vi "Set TDMS logfile.vi"(7 "TDMS Module Alias":string, 8 "log name":string, 9 "Log Directory":string, 10 "Config File Save Path":path, 11 "Config File Path":path) -> (0 "error out":errorcluster)   [LabVIEW 2014]
doc: "Update the log file a TDMS module will write to"
uses:
  <vilib>/NI/DCAF/Modules/TDMS Datalogger/configuration/TDMS datalogger configuration.lvclass
  <vilib>/NI/DCAF/Modules/TDMS Datalogger/configuration/TDMS datalogger configuration.lvclass/TDMS datalogger configuration.ctl
  <vilib>/NI/Configuration Framework/tree serializer/NISE_CEF_TreeSerializer.lvlib
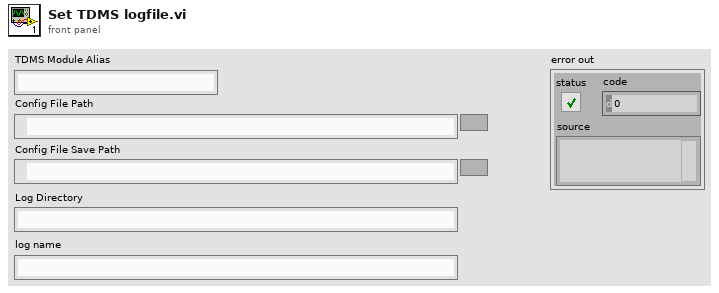
[diagram p1: front panel]
types:
  T1 = typedef "NISE_CEF_TreeSerializer.lvlib/base file format.ctl" = cluster{"version":string, "data":string}
  T2 = typedef "NISE_CEF_TreeSerializer.lvlib/flat hierarchy.ctl" = cluster{"hierarchy structure":T3, "instance data":T5[]}
  T3 = typedef "NISE_CEF_TreeSerializer.lvlib/full hierarchy.ctl" = cluster{"root":string, "hierarchy":T4[]}
  T4 = typedef "NISE_CEF_TreeSerializer.lvlib/hierarchy element.ctl" = cluster{"current node":string, "children":string[]}
  T5 = typedef "NISE_CEF_TreeSerializer.lvlib/instance data.ctl" = cluster{"ID":string, "Alias":string, "class":string, "version":string, "data":string}
  T6 = typedef "NISE_CEF_TreeSerializer.lvlib/memory hierarchy.ctl" = cluster{"hierarchy structure":T3, "instance data":refnum<class "NISE_CEF_serializable configuration.lvclass">[]}
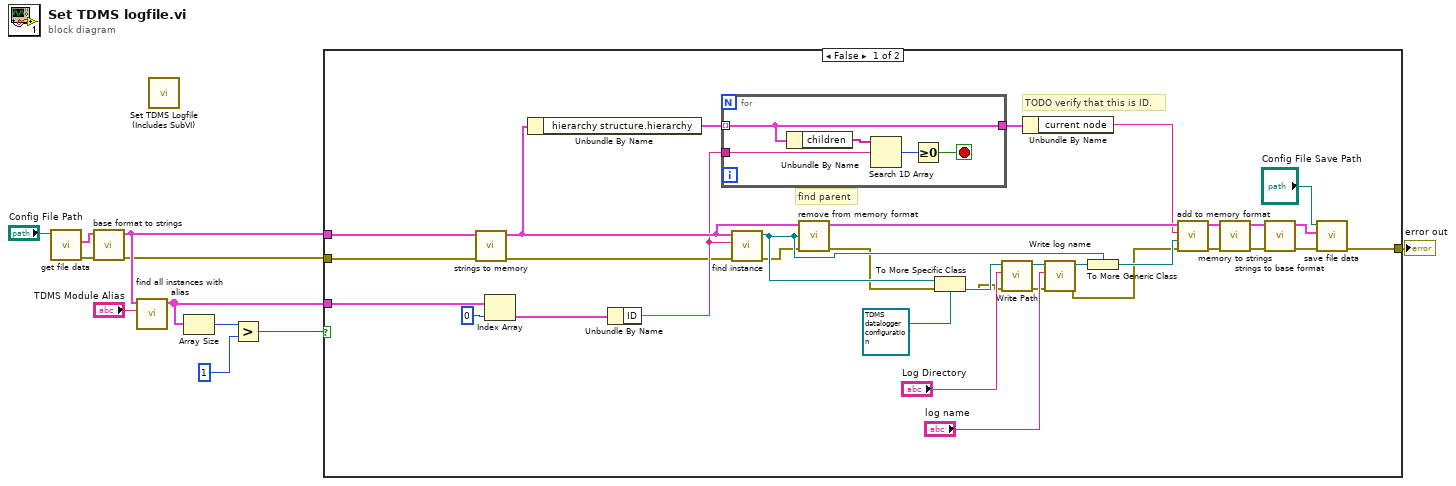
[diagram p0: block diagram]
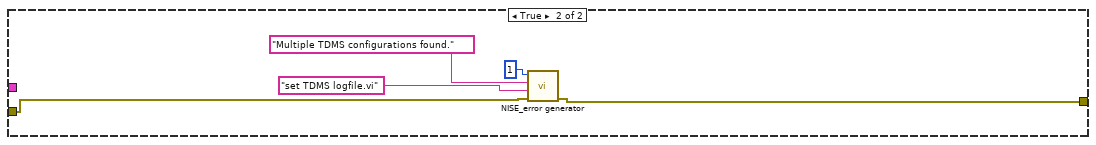
[diagram p2: hidden frame]
diagram:
  n1 = call <vilib>:"get file data.vi"("Path"="Config File Path") -> ("error out"=w11:errorcluster, "format"=w10:T1)  [unwired: 9 in]
  n2 = call <vilib>:"base format to strings.vi"("error in"=w11, "format"=w10) -> ("error out"=w5:errorcluster, "data"=w7:T2)  [unwired: 8 in]
  n3 = call <vilib>:"find all instances with alias.vi"("Alias"="TDMS Module Alias", "flat hierarchy"=w7) -> ("instance data"=w4:T5[])  [unwired: 9 in]
  n4 = call "Set TDMS Logfile (Includes SubVI).vi"() -> ()  [unwired: 12 in]
  n5 = Array Size(array=w4) -> (size(s)=w3:i32)
  n6 = Greater?(x=w3, y=1) -> (0:w1:bool)
  n7 = case shown="False" w1 {
    tunnel: w7 -> [w40 _]
    tunnel: [w19 w50] -> w6
    tunnel: w5 -> [w17 w51]
    tunnel: w4 -> [w12 _]
    frame False {
      # "TODO verify that this is ID."
      # "find parent"
      n8 = call <vilib>:"strings to memory.vi"("error in"=w17, "1.0.0"=w40) -> ("error out"=w16:errorcluster, "memory hierarchy"=w26:T6)  [unwired: 8 in]
      n9 = Index Array(array=w12, index=0) -> (element=w41:T5)
      n10 = Unbundle By Name(w26) -> ("hierarchy structure.hierarchy"=w25:T4[])
      n11 = Unbundle By Name(w41) -> ("ID"=w24:string)
      n12 = for {
        tunnel: w25 -> [w47] mode=indexing
        tunnel: w24 -> [w48]
        tunnel: [w47] -> w23
        stop <- w45 stop-if-true
        n13 = Unbundle By Name(w47) -> ("children"=w49:string[])
        n14 = Search 1D Array(1D array=w49, element=w48) -> (index of element=w46:i32)  [unwired: 1 in]
        n15 = Greater Or Equal To 0?(x=w46) -> (x >= 0?=w45:bool)
      }
      n16 = call <vilib>:"find instance.vi"("error in"=w16, "ID"=w24, "memory hierarchy"=w26) -> ("error out"=w14:errorcluster, "configuration"=w28:refnum<class "NISE_CEF_serializable configuration.lvclass">)  [unwired: 7 in]
      n17 = call <vilib>:"remove from memory format.vi"("error in"=w14, "NISE_CEF_serializable configuration in"=w28, "memory hierarchy in"=w26) -> ("error out"=w13:errorcluster, "memory hierarchy out"=w27:T6)  [unwired: 7 in]
      n18 = To More Specific Class(target class=refnum<class "TDMS datalogger configuration.lvclass"> refnum ("TDMS datalogger configuration"), reference=w28, error in=w13) -> (specific class reference=w39:refnum<class "TDMS datalogger configuration.lvclass">, error out=w35:errorcluster)
      n19 = call <vilib>:"Write Path.vi"("error in (no error)"=w35, "Log Directory"="Log Directory", "TDMS datalogger configuration in"=w39) -> ("error out"=w34:errorcluster, "TDMS datalogger configuration out"=w37:refnum<class "TDMS datalogger configuration.lvclass">)  [unwired: 7 in]
      n20 = Unbundle By Name(w23) -> ("current node"=w22:string)
      n21 = call <vilib>:"Write log name.vi"("error in (no error)"=w34, "log name"="log name", "TDMS datalogger configuration in"=w37) -> ("error out"=w15:errorcluster, "TDMS datalogger configuration out"=w33:refnum<class "TDMS datalogger configuration.lvclass">)  [unwired: 7 in]
      n22 = To More Generic Class(target class=w28, reference=w33) -> (generic class reference=w29:refnum<class "NISE_CEF_serializable configuration.lvclass">)
      n23 = call <vilib>:"add to memory format.vi"("error in"=w15, "NISE_CEF_serializable configuration in"=w29, "parent ID"=w22, "memory hierarchy in"=w27) -> ("error out"=w30:errorcluster, "memory hierarchy out"=w31:T6)  [unwired: 6 in]
      n24 = call <vilib>:"memory to strings.vi"("error in"=w30, "memory hierarchy"=w31) -> ("error out"=w20:errorcluster, "1.0.0"=w21:T2)  [unwired: 8 in]
      n25 = call <vilib>:"strings to base format.vi"("error in"=w20, "1.0.0"=w21) -> ("error out"=w44:errorcluster, "format"=w43:T1)  [unwired: 8 in]
      n26 = call <vilib>:"save file data.vi"("error in"=w44, "format"=w43, "Path"="Config File Save Path") -> ("error out"=w19:errorcluster)  [unwired: 8 in]
    }
    frame True {
      n27 = call <vilib>:"NISE_error generator.vi"("error in"=w51, "source"="set TDMS logfile.vi", "append error message"="Multiple TDMS configurations found.", "error code (0)"=1) -> ("error out"=w50:errorcluster)  [unwired: 5 in]
    }
  }
  "error out" <- w6
